vi "Hemisphere V104 VISA IO.vi"(7 "Sys Msg Queue":refnum<queue>, 8 "error in (no error)":errorcluster, 11 "Enabled?":bool) -> (0 "error out":errorcluster)   [LabVIEW 2019]
doc: "This VI expects a GPS data source on the configured RS232 port. The GPS data should contain the $GPGGA sentence in a standard NMEA ASCII stream. \n\nDefault Settings:\nEnabled - FALSE\nVISA Resource: ASRL4::INSTR\nBaud Rate: 9600\nSerial Port Settings: 8n1"
uses:
  Globals and Definitions/System Message.ctl
  Globals and Definitions/Serial - Settings.ctl
  Globals and Definitions/Initialization Globals.vi
  Globals and Definitions/RT Globals RD v1.0.vi
panel:
  in  "Serial Settings":T1={"baud rate"=9600, "data bits"=8, "parity"=enum."None", "stop bits"=10, "flow control"=0} {"flow control" items=["None"=0, "XON/XOFF"=1, "RTS/CTS"=2, "DTR/DSR"=4]; "stop bits" items=["1.0"=10, "1.5"=15, "2.0"=20]; "data bits" min=5 max=8 step=1; "baud rate" items=["75"=75, "110"=110, "134"=134, "150"=150, "300"=300, "600"=600, "1200"=1200, "1800"=1800, "2400"=2400, "4800"=4800, "7200"=7200, "9600"=9600, "14400"=14400, "19200"=19200, "28800"=28800, "38400"=38400, "56000"=56000, "57600"=57600, "115200"=115200, "128000"=128000, "230400"=230400]}
  in  "VISA resource name":refnum<visa-resource-name>="ASRL4::INSTR"
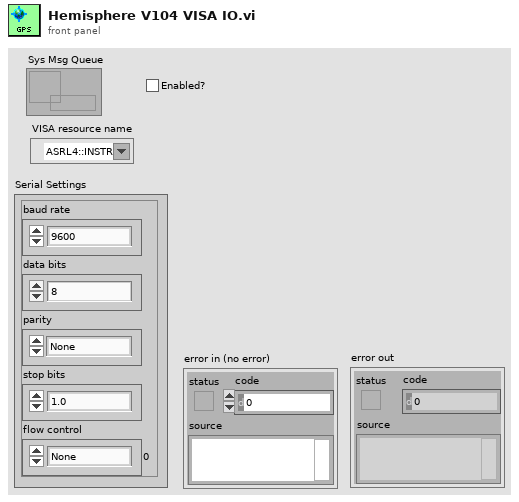
[diagram p1: front panel]
types:
  T1 = typedef "Serial - Settings.ctl" = cluster{"baud rate":u32, "data bits":u16, "parity":enum16{"None", "Odd", "Even", "Mark", "Space"}, "stop bits":u16, "flow control":u16}
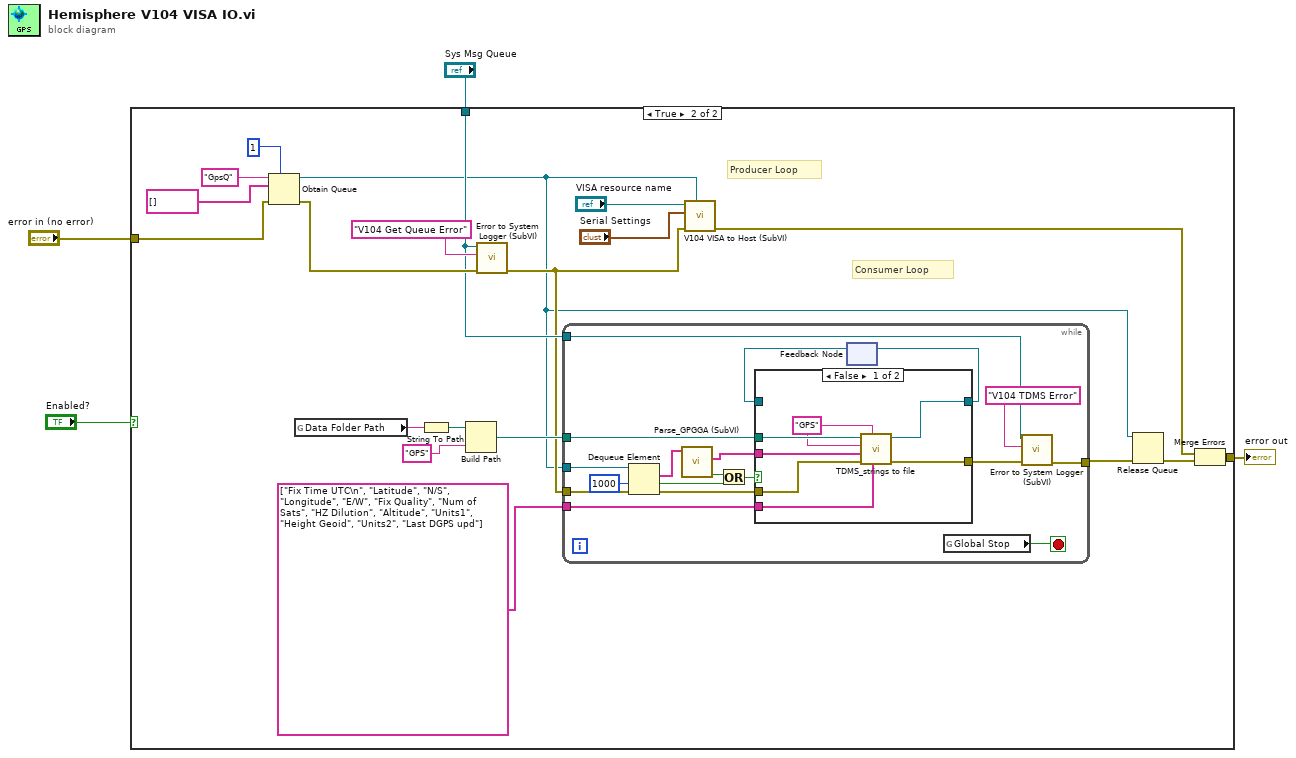
[diagram p0: block diagram]
diagram:
  n1 = case shown="True" "Enabled?" {
    tunnel: [w5 w25] -> w4
    tunnel: "Sys Msg Queue" -> [_ w14]
    tunnel: "error in (no error)" -> [w5 w6]
    frame False {
    }
    frame True {
      # "Consumer Loop"
      # "Producer Loop"
      n2 = Obtain Queue(max queue size (-1, unlimited)=1, name (unnamed)="GpsQ", element data type=string[] [], error in (no error)=w6) -> (queue out=w8:refnum<queue>, error out=w16:errorcluster)  [unwired: 1 in, 1 out]
      n3 = global read "Initialization Globals.vi" "Data Folder Path"() -> (w20:string)
      n4 = String To Path(string=w20) -> (path=w19:path)
      n5 = Build Path(base path=w19, name or relative path="GPS") -> (appended path=w17:path)
      n6 = call "Error to System Logger (SubVI).vi"("error in (no error)"=w16, "Message Tag"="V104 Get Queue Error", "Sys Msg Queue"=w14) -> ("error out"=w9:errorcluster)  [unwired: 8 in]
      n7 = while {
        tunnel: w8 -> [w43]
        tunnel: w9 -> [w39]
        tunnel: [w30] -> w23
        tunnel: string[] ["Fix Time UTC\n", "Latitude", "N/S", "Longitude", "E/W", "Fix Quality", "Num of Sats", "HZ Dilution", "Altitude", "Units1", "Height Geoid", "Units2", "Last DGPS upd"] ("Channel Names") -> [w35]
        tunnel: w17 -> [w34]
        tunnel: w14 -> [w26]
        stop <- w28 stop-if-true
        n8 = Dequeue Element(queue=w43, timeout in ms (-1)=1000, error in (no error)=w39) -> (element=w32:string[], timed out?=w37:bool, error out=w38:errorcluster)  [unwired: 1 out]
        n9 = call "Parse_GPGGA (SubVI).vi"("Array"=w32) -> ("GPGGA?"=w31:bool, "GPGGA array"=w33:string[])  [unwired: 7 in]
        n10 = Or(x=w31, y=w37) -> (x .or. y?=w36:bool)
        n11 = feedback #1() -> (w40:refnum<k34>)  [unwired: 1 in]
        n12 = case shown="False" w36 {
          tunnel: w33 -> [w49 _]
          tunnel: w34 -> [w50 _]
          tunnel: [w48 w52] -> w41
          tunnel: w40 -> [_ w52]
          tunnel: w38 -> [w47 w51]
          tunnel: [w46 w51] -> w29
          tunnel: w35 -> [w44 _]
          frame False {
            w45 = "GPS" ("group name in (Untitled)")
            n13 = call "TDMS_strings to file.vi"("Channel Names"=w44, "Group Name"=w45, "error in (no error)"=w47, "Data"=w49, "Measurement"=w45, "Base path"=w50) -> ("error out"=w46:errorcluster, "file out"=w48:refnum<k34>)  [unwired: 4 in]
          }
          frame True {
          }
        }
        n14 = feedback-in #1(w41) -> ()
        n15 = global read "RT Globals RD v1.0.vi" "Global Stop"() -> (w28:bool)
        n16 = call "Error to System Logger (SubVI).vi"("error in (no error)"=w29, "Message Tag"="V104 TDMS Error", "Sys Msg Queue"=w26) -> ("error out"=w30:errorcluster)  [unwired: 8 in]
      }
      n17 = call "V104 VISA to Host (SubVI).vi"("Serial Queue In"=w8, "error in (no error)"=w9, "Serial Settings"="Serial Settings", "VISA resource name"="VISA resource name") -> ("error out"=w12:errorcluster)  [unwired: 7 in]
      n18 = Release Queue(queue=w8, error in (no error)=w23) -> (error out=w13:errorcluster)  [unwired: 1 in, 2 out]
      n19 = Merge Errors(w12, w13) -> (w25:errorcluster)
    }
  }
  "error out" <- w4
